vi "ADIS16470 Read.vi"(8 "error in (no error)":errorcluster, 11 "ADIS16470DevRef":T2={"DevStatus"={"status"=FALSE, "code"=0, "source"=""}, "Hardware Config"={"SPI Clock Rate (Hz)"=0.0, "IMU SPI Mode (3)"=enum."Mode 0 (Clk Idle Low,Sample on Leading)", "IMU Reset Pin"=enum."DIO 0", "IMU SPI Bus"=enum."SPI On-Board, CS0", "IMU Data Ready Pin"=enum."DIO 0", "Stall Config"={"Pow2BytesPerRead"=255, "StallTicks"=640, "CsToSclkTicks"=5}}, "Calibration Complete"=refnum, "Status Reference"=refnum, "Data Reference"=refnum, "Sychronous Process VI"=refnum, "Cmd FIFO"=refnum, "Source"={"DevStatus"={"status"=FALSE, "code"=0, "source"=""}, "AnalogTriggerMode?"=FALSE, "DigitalMode"={"DIO Channel"=enum."Disabled"}, "AnalogTriggerMode"={"AnalogTriggerIndex"=enum."Trig 0", "OutputType"=enum."InWindow"}}, "Data FIFO"=refnum, "Calibration Time (ms)"=5, "Data Reference"=refnum}) -> (0 "error out":errorcluster, 1 "ADIS16470 Buffer":T1[](array[typedef]), 2 "ADIS16470 Value":T1, 3 "ADIS16470DevRef":T2={"DevStatus"={"status"=FALSE, "code"=0, "source"=""}, "Hardware Config"={"SPI Clock Rate (Hz)"=0.0, "IMU SPI Mode (3)"=enum."Mode 0 (Clk Idle Low,Sample on Leading)", "IMU Reset Pin"=enum."DIO 0", "IMU SPI Bus"=enum."SPI On-Board, CS0", "IMU Data Ready Pin"=enum."DIO 0", "Stall Config"={"Pow2BytesPerRead"=255, "StallTicks"=640, "CsToSclkTicks"=5}}, "Calibration Complete"=refnum, "Status Reference"=refnum, "Data Reference"=refnum, "Sychronous Process VI"=refnum, "Cmd FIFO"=refnum, "Source"={"DevStatus"={"status"=FALSE, "code"=0, "source"=""}, "AnalogTriggerMode?"=FALSE, "DigitalMode"={"DIO Channel"=enum."Disabled"}, "AnalogTriggerMode"={"AnalogTriggerIndex"=enum."Trig 0", "OutputType"=enum."InWindow"}}, "Data FIFO"=refnum, "Calibration Time (ms)"=5, "Data Reference"=refnum})   [LabVIEW 2025]
doc: "Read the most recent X, Y, and Z angles of the IMU. If configured at open, also return a buffer of recent points."
uses:
  <vilib>/Rock Robotics/WPI/ThirdParty/ADI/ADIS16470/Typedef/ADIS16470 Device Reference.ctl
  <vilib>/Rock Robotics/WPI/ThirdParty/ADI/ADIS16470/Typedef/ADIS16470 Hardware Configuration.ctl
  <vilib>/Rock Robotics/WPI/SPI/WPI_SPIMode.ctl
  <vilib>/Rock Robotics/SystemInterfaces/DIO/FPGA_DIOChannel.ctl
  <vilib>/Rock Robotics/SystemInterfaces/spilib/spi_bus.ctl
  <vilib>/Rock Robotics/WPI/ThirdParty/ADI/ADIS16470/Typedef/ADIS16470 Status.ctl
  <vilib>/Rock Robotics/WPI/ThirdParty/ADI/ADIS16470/Typedef/ADIS16470 Data.ctl
  <vilib>/Rock Robotics/WPI/ThirdParty/ADI/ADIS16470/Typedef/ADIS16470 Process.ctl
  <vilib>/Rock Robotics/WPI/ThirdParty/ADI/ADIS16470/Typedef/ADIS16470 Command Type.ctl
  <vilib>/Rock Robotics/SystemInterfaces/CounterEncoderSourceConvertion/FPGA_CounterEncoderSourceConvertionLVSourceType.ctl
  <vilib>/Rock Robotics/SystemInterfaces/DIO/FPGA_DIODigitalSourceChannel.ctl
  <vilib>/Rock Robotics/SystemInterfaces/AnalogTrigger/FPGA_AnalogTriggerIndex.ctl
  <vilib>/Rock Robotics/SystemInterfaces/AnalogTrigger/FPGA_AnalogTriggerOutType.ctl
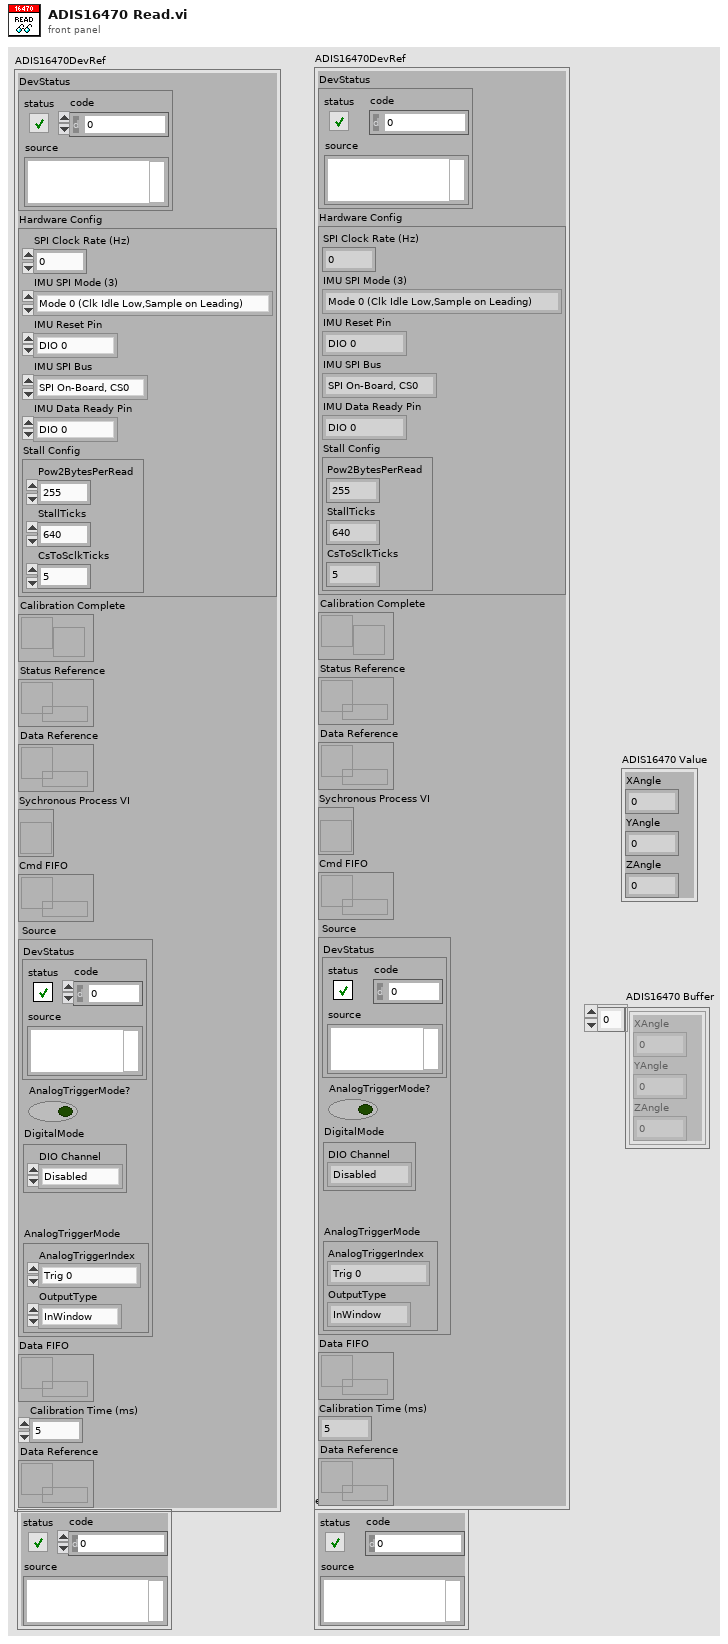
[diagram p1: front panel]
types:
  T1 = typedef "ADIS16470 Data.ctl" = cluster{"XAngle":dbl, "YAngle":dbl, "ZAngle":dbl}
  T2 = typedef "ADIS16470 Device Reference.ctl" = cluster{"DevStatus":errorcluster, "Hardware Config":T3, "Calibration Complete":refnum<notifier>, "Status Reference":refnum<data-value>, "Data Reference":refnum<data-value>, "Sychronous Process VI":T7, "Cmd FIFO":refnum<k33>, "Source":T8, "Data FIFO":refnum<k33>, "Calibration Time (ms)":u32, "Data Reference":refnum<data-value>}
  T3 = typedef "ADIS16470 Hardware Configuration.ctl" = cluster{"SPI Clock Rate (Hz)":dbl, "IMU SPI Mode (3)":T4, "IMU Reset Pin":T5, "IMU SPI Bus":T6, "IMU Data Ready Pin":T5, "Stall Config":cluster{"Pow2BytesPerRead":u8, "StallTicks":u16, "CsToSclkTicks":u8}}
  T4 = typedef "WPI_SPIMode.ctl" = enum16{"Mode 0 (Clk Idle Low,Sample on Leading)", "Mode 1 (Clk Idle Low,Sample on Trailing)", "Mode 2 (Clk Idle High,Sample on Leading)", "Mode 3 (Clk Idle High,Sample on Trailing)"}
  T5 = typedef "FPGA_DIOChannel.ctl" = enum8{"DIO 0", "DIO 1", "DIO 2", "DIO 3", "DIO 4", "DIO 5", "DIO 6", "DIO 7", "DIO 8", "DIO 9", "DIO MXP 0", "DIO MXP 1", "DIO MXP 2", "DIO MXP 3", "DIO MXP 4", "DIO MXP 5", "DIO MXP 6", "DIO MXP 7", "DIO MXP 8", "DIO MXP 9", "DIO MXP 10", "DIO MXP 11", "DIO MXP 12", "DIO MXP 13", "DIO MXP 14", "DIO MXP 15", "SPI Port CS1", "SPI Port CS2", "SPI Port CS3", "SPI Port MISO", "SPI Port MOSI", "Invalid"}
  T6 = typedef "spi_bus.ctl" = enum16{"SPI On-Board, CS0", "SPI On-Board, CS1", "SPI On-Board, CS2", "SPI On-Board, CS3", "SPI MXP", "Invalid"}
  T7 = typedef "ADIS16470 Process.ctl" = refnum<vi>
  T8 = typedef "FPGA_CounterEncoderSourceConvertionLVSourceType.ctl" = cluster{"DevStatus":errorcluster, "AnalogTriggerMode?":bool, "DigitalMode":cluster{"DIO Channel":T9}, "AnalogTriggerMode":cluster{"AnalogTriggerIndex":T10, "OutputType":T11}}
  T9 = typedef "FPGA_DIODigitalSourceChannel.ctl" = enum8{"DIO 0", "DIO 1", "DIO 2", "DIO 3", "DIO 4", "DIO 5", "DIO 6", "DIO 7", "DIO 8", "DIO 9", "DIO MXP 0", "DIO MXP 1", "DIO MXP 2", "DIO MXP 3", "DIO MXP 4", "DIO MXP 5", "DIO MXP 6", "DIO MXP 7", "DIO MXP 8", "DIO MXP 9", "DIO MXP 10", "DIO MXP 11", "DIO MXP 12", "DIO MXP 13", "DIO MXP 14", "DIO MXP 15", "SPI Port CS1", "SPI Port CS2", "SPI Port CS3", "SPI Port MISO", "SPI Port MOSI", "Disabled"}
  T10 = typedef "FPGA_AnalogTriggerIndex.ctl" = enum8{"Trig 0", "Trig 1", "Trig 2", "Trig 3", "Trig 4", "Trig 5", "Trig 6", "Trig 7", "Invalid"}
  T11 = typedef "FPGA_AnalogTriggerOutType.ctl" = enum16{"InWindow", "TriggerState", "Rising", "Falling"}
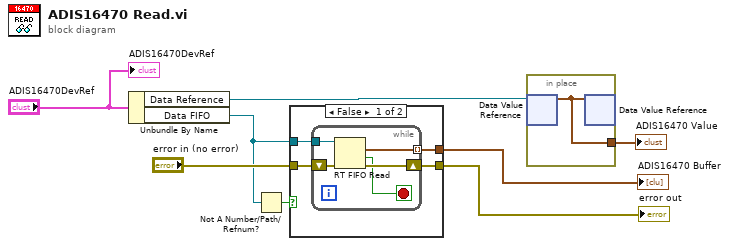
[diagram p0: block diagram]
diagram:
  n1 = Unbundle By Name("ADIS16470DevRef") -> ("Data Reference"=w6:refnum<data-value>, "Data FIFO"=w2:refnum<k33>)
  n2 = Not A Number/Path/Refnum?(number/path/refnum=w2) -> (NaN/Path/Refnum?=w1:bool)
  n3 = case shown="False" w1 {
    tunnel: "error in (no error)" -> [w12 w18]
    tunnel: w2 -> [w11 _]
    tunnel: [w10 w18] -> w5
    tunnel: [w9 _] -> w4
    frame False {
      n4 = while {
        tunnel: w11 -> [w16]
        tunnel: [w13] -> w9 mode=indexing
        shift-right: [w15] -> w10
        shift-left: w12 -> [w17]
        stop <- w14 stop-if-true
        n5 = RT FIFO Read(0:w16, 3:w17) -> (9:w13:T1, 10:w14:bool, 11:w15:errorcluster)  [unwired: 2 in, 2 out]
      }
    }
    frame True {
    }
  }
  "error out" <- w5
  "ADIS16470 Buffer" <- w4
  n6 = in-place {
    in-place-border: [w19] -> w3
    n7 = in-place-dvr #1(w6) -> (w19:T1)  [unwired: 1 out]
    n8 = in-place-dvr #1(w19) -> ()  [unwired: 2 out]
  }
  "ADIS16470 Value" <- w3
  "ADIS16470DevRef" <- "ADIS16470DevRef"
